vi "GEOM_FPA2ReadMode.vi"(9 "Detnumber":i32, 10 "ReadMode":T7 {"amplifiers"."fliped" items=["none", "horizontal", "vertical"]; "amplifiers"."type" items=["LL", "LR", "UL", "UR"]}) -> (2 "output ReadMode":T2 {"Amplifiers"."fliped" items=["none", "horizontal", "vertical"]; "Amplifiers"."type" items=["LL", "LR", "UL", "UR"]})   [LabVIEW 2016]
uses:
  GEOM_ReadMode.ctl
  GEOM_Amplifier.ctl
  GEOM_AmpType.ctl
  GEOM_ROI.ctl
  GEOM_Coords.ctl
  GEOM_FPAReadMode.ctl
panel:
  in  "Case Constant\n(See Context Help)":bool
  in  "roi":T1
  in  "Amplifier":T3={"number"=0, "type"=0, "rotated"=0, "fliped"=0, "FPAcoord"={"xstart"=1, "ystart"=1}, "Physical_size"={"columns"=0, "rows"=0}, "predata"={"columns"=0, "rows"=0}, "postdata"={"columns"=0, "rows"=0}, "Req ROIs"=[], "Corr ROI"=[], "Detnumber"=0, "ampID"="", "discard"=0} {"fliped" items=["none", "horizontal", "vertical"]; "type" items=["LL", "LR", "UL", "UR"]}
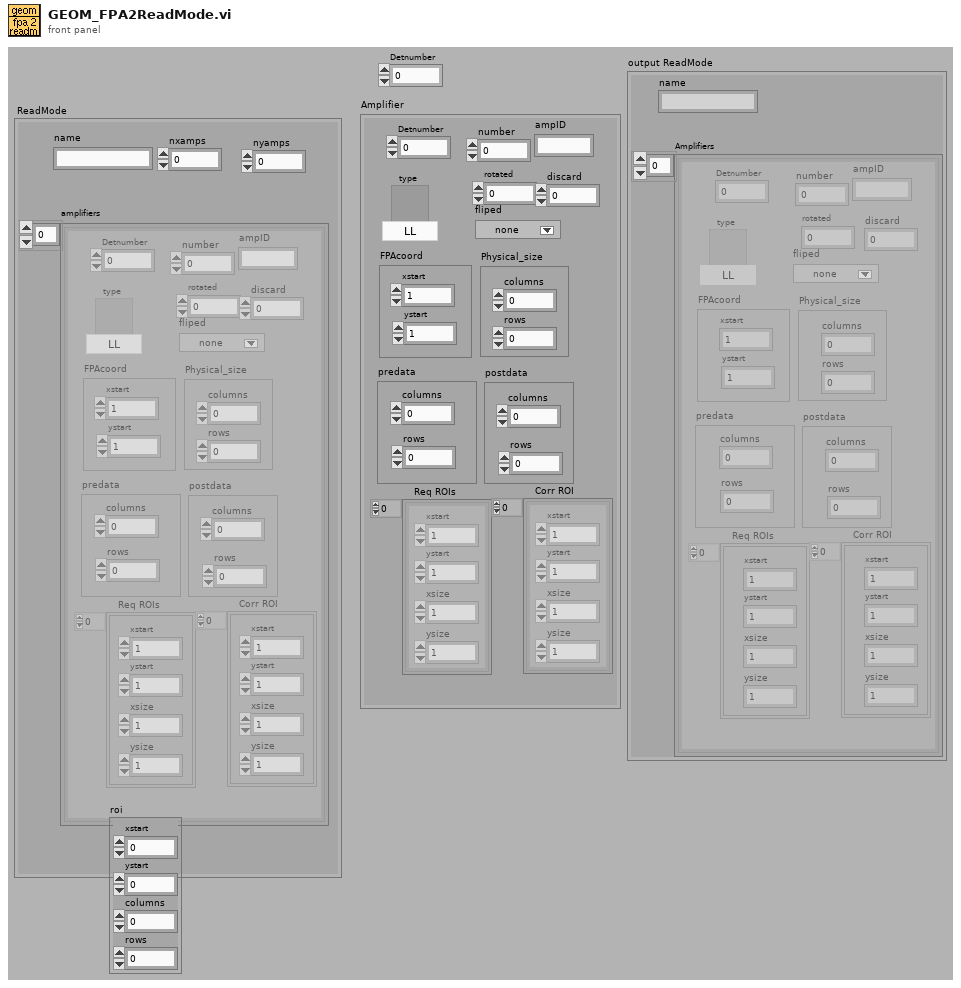
[diagram p1: front panel]
types:
  T1 = cluster{"xstart":u32, "ystart":u32, "columns":u32, "rows":u32}
  T2 = typedef "GEOM_FPAReadMode.ctl" = cluster{"name":string, "Amplifiers":T3[]}
  T3 = typedef "GEOM_Amplifier.ctl" = cluster{"number":i32, "type":T4, "rotated":i16, "fliped":u16, "FPAcoord":cluster{"xstart":i32, "ystart":i32}, "Physical_size":cluster{"columns":i32, "rows":i32}, "predata":cluster{"columns":i32, "rows":i32}, "postdata":cluster{"columns":i32, "rows":i32}, "Req ROIs":T5, "Corr ROI":T5, "Detnumber":i32, "ampID":string, "discard":i32}
  T4 = typedef "GEOM_AmpType.ctl" = u16
  T5 = typedef "GEOM_ROI.ctl" = T6[]
  T6 = typedef "GEOM_Coords.ctl" = cluster{"xstart":u32, "ystart":u32, "xsize":u32, "ysize":u32}
  T7 = typedef "GEOM_ReadMode.ctl" = cluster{"name":string, "amplifiers":T3[], "nxamps":i32, "nyamps":i32}
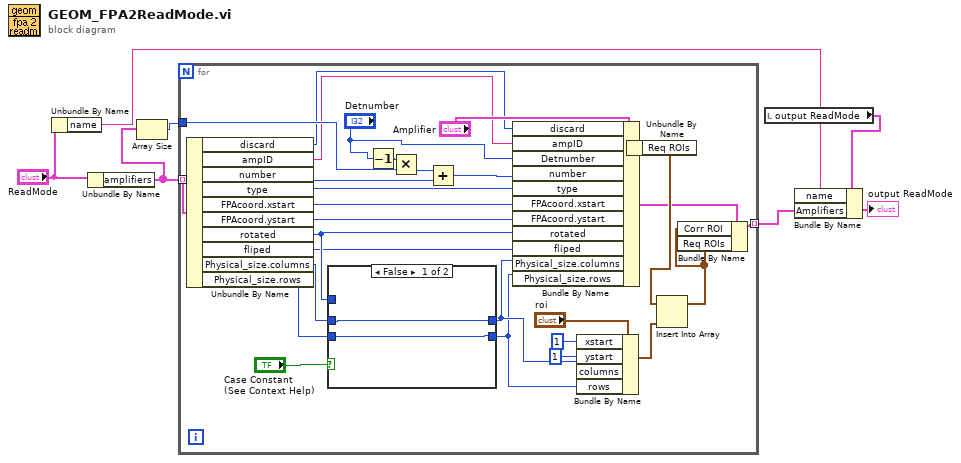
[diagram p0: block diagram]
diagram:
  n1 = Unbundle By Name("ReadMode") -> ("name"=w6:string)
  n2 = Unbundle By Name("ReadMode") -> ("amplifiers"=w4:T3[])
  n3 = Array Size(array=w4) -> (size(s)=w3:i32)
  n4 = for {
    tunnel: w4 -> [w35] mode=indexing
    tunnel: [w18] -> w1 mode=indexing
    tunnel: w3 -> [w13]
    n5 = Unbundle By Name(w35) -> ("discard"=w8:i32, "ampID"=w10:string, "number"=w14:i32, "type"=w34:T4, "FPAcoord.xstart"=w33:i32, "FPAcoord.ystart"=w32:i32, "rotated"=w31:i16, "fliped"=w30:u16, "Physical_size.columns"=w29:i32, "Physical_size.rows"=w28:i32)
    n6 = case shown="False" "Case Constant\n(See Context Help)" {
      tunnel: w31 -> [_ w42]
      tunnel: w29 -> [w37 w41]
      tunnel: w28 -> [w36 w40]
      tunnel: [w37 w39] -> w23
      tunnel: [w36 w38] -> w22
      frame False {
      }
      frame True {
        n7 = case shown="-270, -90, 90, 270" w42 {
          tunnel: w41 -> [w44 w46]
          tunnel: w40 -> [w43 w45]
          tunnel: [w43 w46] -> w39
          tunnel: [w44 w45] -> w38
          frame -270, -90, 90, 270 {
          }
          frame 0, Default {
          }
        }
      }
    }
    n8 = Decrement(x="Detnumber") -> (x-1=w12:i32)
    n9 = Multiply(x=w12, y=w13) -> (x*y=w15:i32)
    n10 = Add(x=w15, y=w14) -> (x+y=w11:i32)
    n11 = Bundle By Name(cluster="Amplifier", "discard"=w8, "ampID"=w10, "Detnumber"="Detnumber", "number"=w11, "type"=w34, "FPAcoord.xstart"=w33, "FPAcoord.ystart"=w32, "rotated"=w31, "fliped"=w30, "Physical_size.columns"=w23, "Physical_size.rows"=w22) -> (w19:T3)
    n12 = Bundle By Name(cluster="roi", "xstart"=u32 1, "ystart"=u32 1, "columns"=w23, "rows"=w22) -> (w20:T1)
    n13 = Unbundle By Name("Amplifier") -> ("Req ROIs"=w21:T5)
    n14 = Insert Into Array(array=w21, new element=w20) -> (w17:T5)  [unwired: 1 in]
    n15 = Bundle By Name(cluster=w19, "Corr ROI"=w17, "Req ROIs"=w17) -> (w18:T3)
  }
  n16 = local read "output ReadMode"() -> (w2:T2)
  n17 = Bundle By Name(cluster=w2, "name"=w6, "Amplifiers"=w1) -> (→"output ReadMode":T2)
